vi "Blend.vi"(7 "Source Name in":string, 8 "error in (no error)":errorcluster, 9 "Source Enqueuer":refnum<class "Message Enqueuer.lvclass">, 10 "Sample to Blend in":refnum<class "Sample.lvclass">, 11 "Capillary Line in":refnum<class "Capillary Line.lvclass">) -> (0 "error out":errorcluster, 2 "Source Name":string, 3 "Capillary Line out":refnum<class "Capillary Line.lvclass">)   [LabVIEW 2015, in "cRIO-Carbondioxide.lvlib" / "CO2-Actor.lvlib" / "Capillary Line.lvclass"]
uses:
  Capillary Line.lvclass
  subs/Sample/Sample.lvclass
  <vilib>/ActorFramework/Message Enqueuer/Message Enqueuer.lvclass
  Valve/Valve.lvclass
  Capillary Line.lvclass/Capillary Line.ctl
  CO2 Actor Messages/Ping Msg/Ping Msg.lvclass/Ping Msg.ctl
  <vilib>/ActorFramework/Message Enqueuer/Message Enqueuer.lvclass/Message Enqueuer.ctl
  <vilib>/ActorFramework/Message Enqueuer/Enqueue.vi
  <vilib>/ActorFramework/Message Priority Queue/Priority Enqueue.vi
  CO2 Actor/CO2 Actor.lvclass
  CO2 Actor Messages/Ping Msg/Ping Msg.lvclass
  <vilib>/ActorFramework/Actor/Actor.lvclass
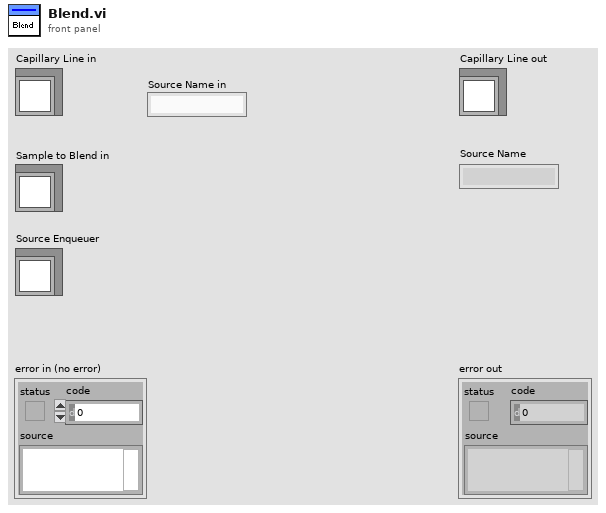
[diagram p1: front panel]
types:
  T1 = typedef "Sample Container.ctl" = cluster{"Sample In":refnum<k21>, "Sample Name":refnum<k21>, "Ti Cathode":refnum<k21>, "SampleQ":refnum<queue>}
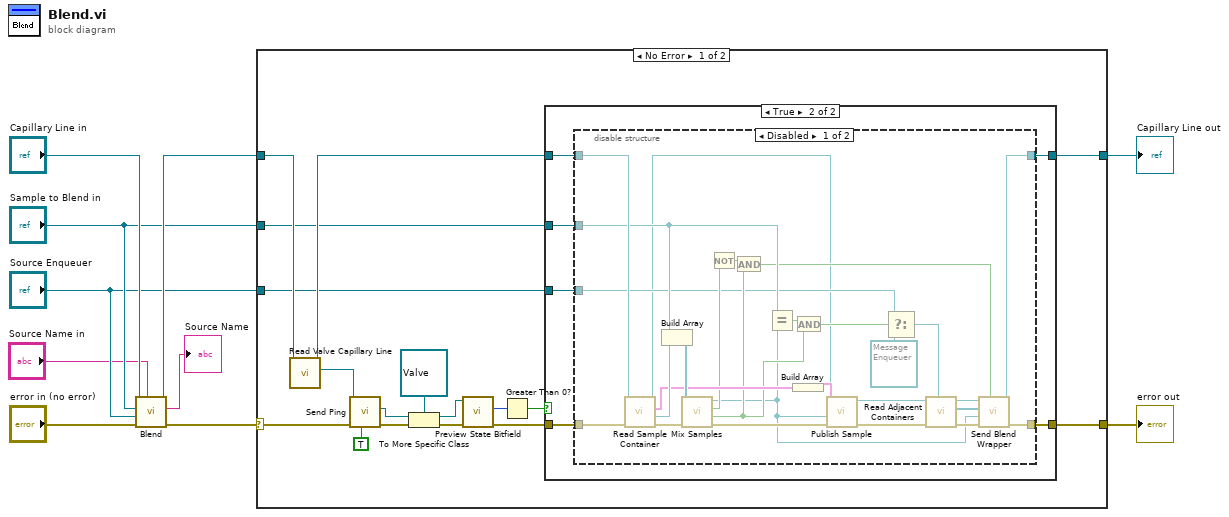
[diagram p0: block diagram]
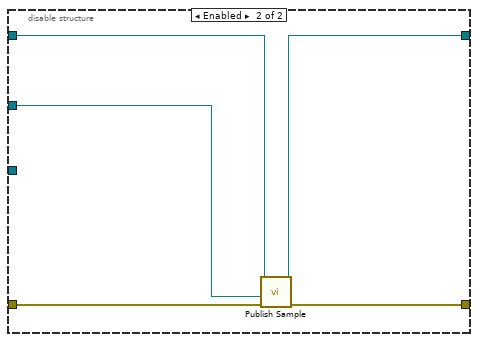
[diagram p3: hidden frame]
diagram:
  n1 = call-parent "Blend.vi"("Source Name in"="Source Name in", "error in (no error)"="error in (no error)", "Source Enqueuer"="Source Enqueuer", "Sample to Blend in"="Sample to Blend in", "CO2 Actor in"="Capillary Line in") -> ("error out"=w6:errorcluster, "Source Name"=→"Source Name":string, "CO2 Actor out"=w7:refnum<class "Capillary Line.lvclass">)  [unwired: 4 in]
  n2 = case shown="No Error" w6 {
    selector: w6 -> [w26 w68]
    tunnel: w7 -> [w27 w69]
    tunnel: [w15 w69] -> w5
    tunnel: "Sample to Blend in" -> [w14 _]
    tunnel: "Source Enqueuer" -> [w13 _]
    tunnel: [w11 w68] -> w2
    frame No Error {
      n3 = call "Read Valve Capillary Line.vi"("Capillary Line in"=w27) -> ("Actor Framework:Message Enqueuer"=w25:refnum<class "Message Enqueuer.lvclass">, "Capillary Line out"=w16:refnum<class "Capillary Line.lvclass">)  [unwired: 9 in]
      n4 = call "Send Ping.vi"("Return Self (F)"=TRUE, "error in (no error)"=w26, "Message Enqueuer"=w25) -> ("error out"=w21:errorcluster, "Actor out"=w23:refnum<class "Actor.lvclass">)  [unwired: 5 in, 2 out]
      n5 = To More Specific Class(target class=refnum<class "Valve.lvclass"> refnum ("Valve.lvclass"), reference=w23, error in=w21) -> (specific class reference=w19:refnum<class "Valve.lvclass">, error out=w20:errorcluster)
      n6 = call "Preview State Bitfield.vi"("error in (no error)"=w20, "Valve in"=w19) -> ("error out"=w17:errorcluster, "State Bitfield"=w18:u16)  [unwired: 7 in, 1 out]
      n7 = Greater Than 0?(x=w18) -> (x > 0?=w12:bool)
      n8 = case shown="True" w12 {
        tunnel: w17 -> [w28 w35]
        tunnel: w16 -> [w29 w34]
        tunnel: [w29 w30] -> w15
        tunnel: w14 -> [_ w33]
        tunnel: w13 -> [_ w32]
        tunnel: [w28 w31] -> w11
        frame False {
        }
        frame True {
          n9 = disable-structure shown="Disabled" {
            disable-tunnel: w35 -> [w62 w63]
            disable-tunnel: w34 -> [w58 w65]
            disable-tunnel: w33 -> [w52 w67]
            disable-tunnel: w32 -> [w46 _]
            disable-tunnel: [w38 w66] -> w31
            disable-tunnel: [w36 w64] -> w30
            frame Disabled {
              n10 = call "Read Sample Container.vi"("error in (no error)"=w62, "Capillary Line in"=w58) -> ("error out"=w61:errorcluster, "Sample"=w60:refnum<class "Sample.lvclass">, "Container"=w54:T1, "Capillary Line out"=w37:refnum<class "Capillary Line.lvclass">)  [unwired: 6 in]
              n11 = Build Array(w52, w60) -> (w59:refnum<class "Sample.lvclass">[])
              n12 = call "Mix Samples.vi"("error in (no error)"=w61, "Samples In"=w59) -> ("error out"=w57:errorcluster, "is clean?"=w48:bool, "Empty Samples present?"=w50:bool, "Sample out"=w39:refnum<class "Sample.lvclass">)  [unwired: 6 in]
              n13 = Not(x=w50) -> (.not. x?=w51:bool)
              n14 = And(x=w51, y=w48) -> (x .and. y?=w42:bool)
              n15 = Equal?(x=w52, y=w39) -> (x = y?=w49:bool)
              n16 = Build Array(w54) -> (w53:T1[])
              n17 = And(x=w49, y=w48) -> (x .and. y?=w47:bool)
              n18 = call "Publish Sample.vi"("error in (no error)"=w57, "Sample"=w39, 10:w53, "Capillary Line in"=w37) -> ("error out"=w56:errorcluster, "Capillary Line in 2"=w55:refnum<class "Capillary Line.lvclass">)  [unwired: 6 in]
              n19 = Select(t=w46, s=w47, f=refnum<class "Message Enqueuer.lvclass"> refnum) -> (s? t:f=w41:refnum<class "Message Enqueuer.lvclass">)
              n20 = call "Read Adjacent Containers.vi"("Exclude Source"=w41, "error in (no error)"=w56, "Capillary Line in"=w55) -> ("error out"=w44:errorcluster, "Adjacent Containers"=w40:refnum<class "Message Enqueuer.lvclass">[], "Capillary Line out"=w43:refnum<class "Capillary Line.lvclass">)  [unwired: 6 in]
              n21 = call-dynamic "Send Blend Wrapper.vi"("Include Source EnQr (T)"=w42, "error in (no error)"=w44, "Sample to Blend"=w39, "Send to"=w40, "CO2 Actor in"=w43) -> ("error out"=w38:errorcluster, "CO2 Actor out"=w36:refnum<class "Capillary Line.lvclass">)  [unwired: 5 in]
            }
            frame Enabled {
              n22 = call "Publish Sample.vi"("error in (no error)"=w63, "Sample"=w67, "Capillary Line in"=w65) -> ("error out"=w66:errorcluster, "Capillary Line in 2"=w64:refnum<class "Capillary Line.lvclass">)  [unwired: 7 in]
            }
          }
        }
      }
    }
    frame Error {
    }
  }
  "error out" <- w2
  "Capillary Line out" <- w5
